vi "Nest Msg Send.vi"(7 "Self Actor":refnum<class "LVCAM.lvclass">, 8 "Alias":string, 9 "Priority?":bool, 10 "Msg":refnum<class "Msg.lvclass">) -> (0 "error out":errorcluster, 2 "Alias found?":bool)   [LabVIEW 2021, in "LVCAM.lvlib" / "Self Actor.lvclass"]
uses:
  Self Actor.lvclass
  Msg/Msg.lvclass
  LVCAM/LVCAM.lvclass
  Msg Q/Msg Q.lvclass
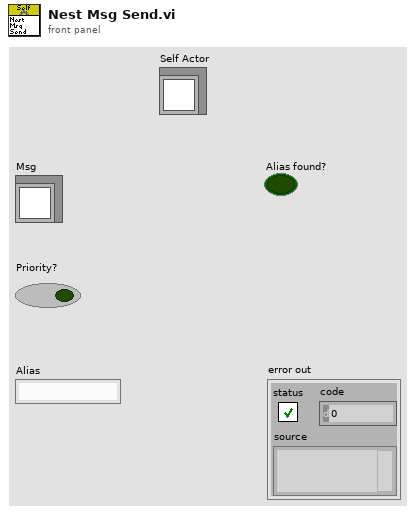
[diagram p1: front panel]
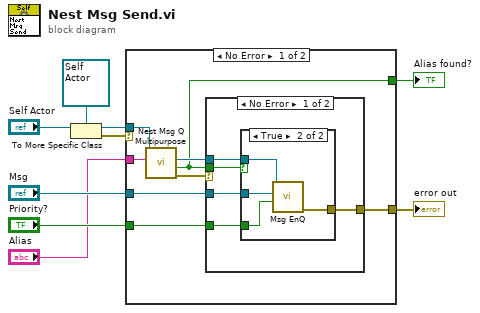
[diagram p0: block diagram]
diagram:
  n1 = To More Specific Class(target class=refnum<class "Self Actor.lvclass"> refnum ("LVCAM.lvlib:Self Actor.lvclass"), reference="Self Actor") -> (specific class reference=w5:refnum<class "Self Actor.lvclass">, error out=w3:errorcluster)  [unwired: 1 in]
  n2 = case shown="No Error" w3 {
    selector: w3 -> [_ w28]
    tunnel: [w17 w28] -> w9
    tunnel: "Msg" -> [w16 _]
    tunnel: "Priority?" -> [w15 _]
    tunnel: w5 -> [w12 _]
    tunnel: "Alias" -> [w13 _]
    tunnel: [w10 _] -> w1
    frame No Error {
      n3 = call "Nest Msg Q Multipurpose.vi"("Alias"=w13, "Self Actor in"=w12) -> ("error out"=w14:errorcluster, "Alias found?"=w10:bool, "Nest Msg Q"=w11:refnum<class "Msg Q.lvclass">)  [unwired: 5 in, 2 out]
      n4 = case shown="No Error" w14 {
        selector: w14 -> [_ w27]
        tunnel: [w22 w27] -> w17
        tunnel: w16 -> [w21 _]
        tunnel: w15 -> [w20 _]
        tunnel: w10 -> [w19 _]
        tunnel: w11 -> [w18 _]
        frame No Error {
          n5 = case shown="True" w19 {
            tunnel: [_ w24] -> w22
            tunnel: w21 -> [_ w26]
            tunnel: w20 -> [_ w25]
            tunnel: w18 -> [_ w23]
            frame False {
            }
            frame True {
              n6 = call "Msg EnQ.vi"("Priority?"=w25, "Msg"=w26, "Msg Q in"=w23) -> ("error out"=w24:errorcluster)  [unwired: 8 in]
            }
          }
        }
        frame Error {
          # "#LVCAMError"
        }
      }
    }
    frame Error {
    }
  }
  "error out" <- w9
  "Alias found?" <- w1
